vi "ComparaDataUART.vi"(8 "error in (no error)":errorcluster, 10 "StringIN":string, 11 "XuLyStringUART in":refnum<class "XuLyStringUART.lvclass">) -> (0 "error out":errorcluster, 3 "XuLyStringUART out":refnum<class "XuLyStringUART.lvclass">)   [LabVIEW 2017, in "LibraryGcode.lvlib" / "XuLyStringUART.lvclass"]
uses:
  XuLyStringUART.lvclass
  control/UartTypeDataGet.ctl
  controls/state_board_control.ctl
  XuLyStringUART.lvclass/XuLyStringUART.ctl
  control/UartStatusBusy.ctl
panel:
  out "outPOS":T1
  out "OUTCONFIG":T2
  out "Return State 2":T3=enum."Echo"
  in  "error IN":errorcluster
  out "error out 2":errorcluster
  in  "String IN":string
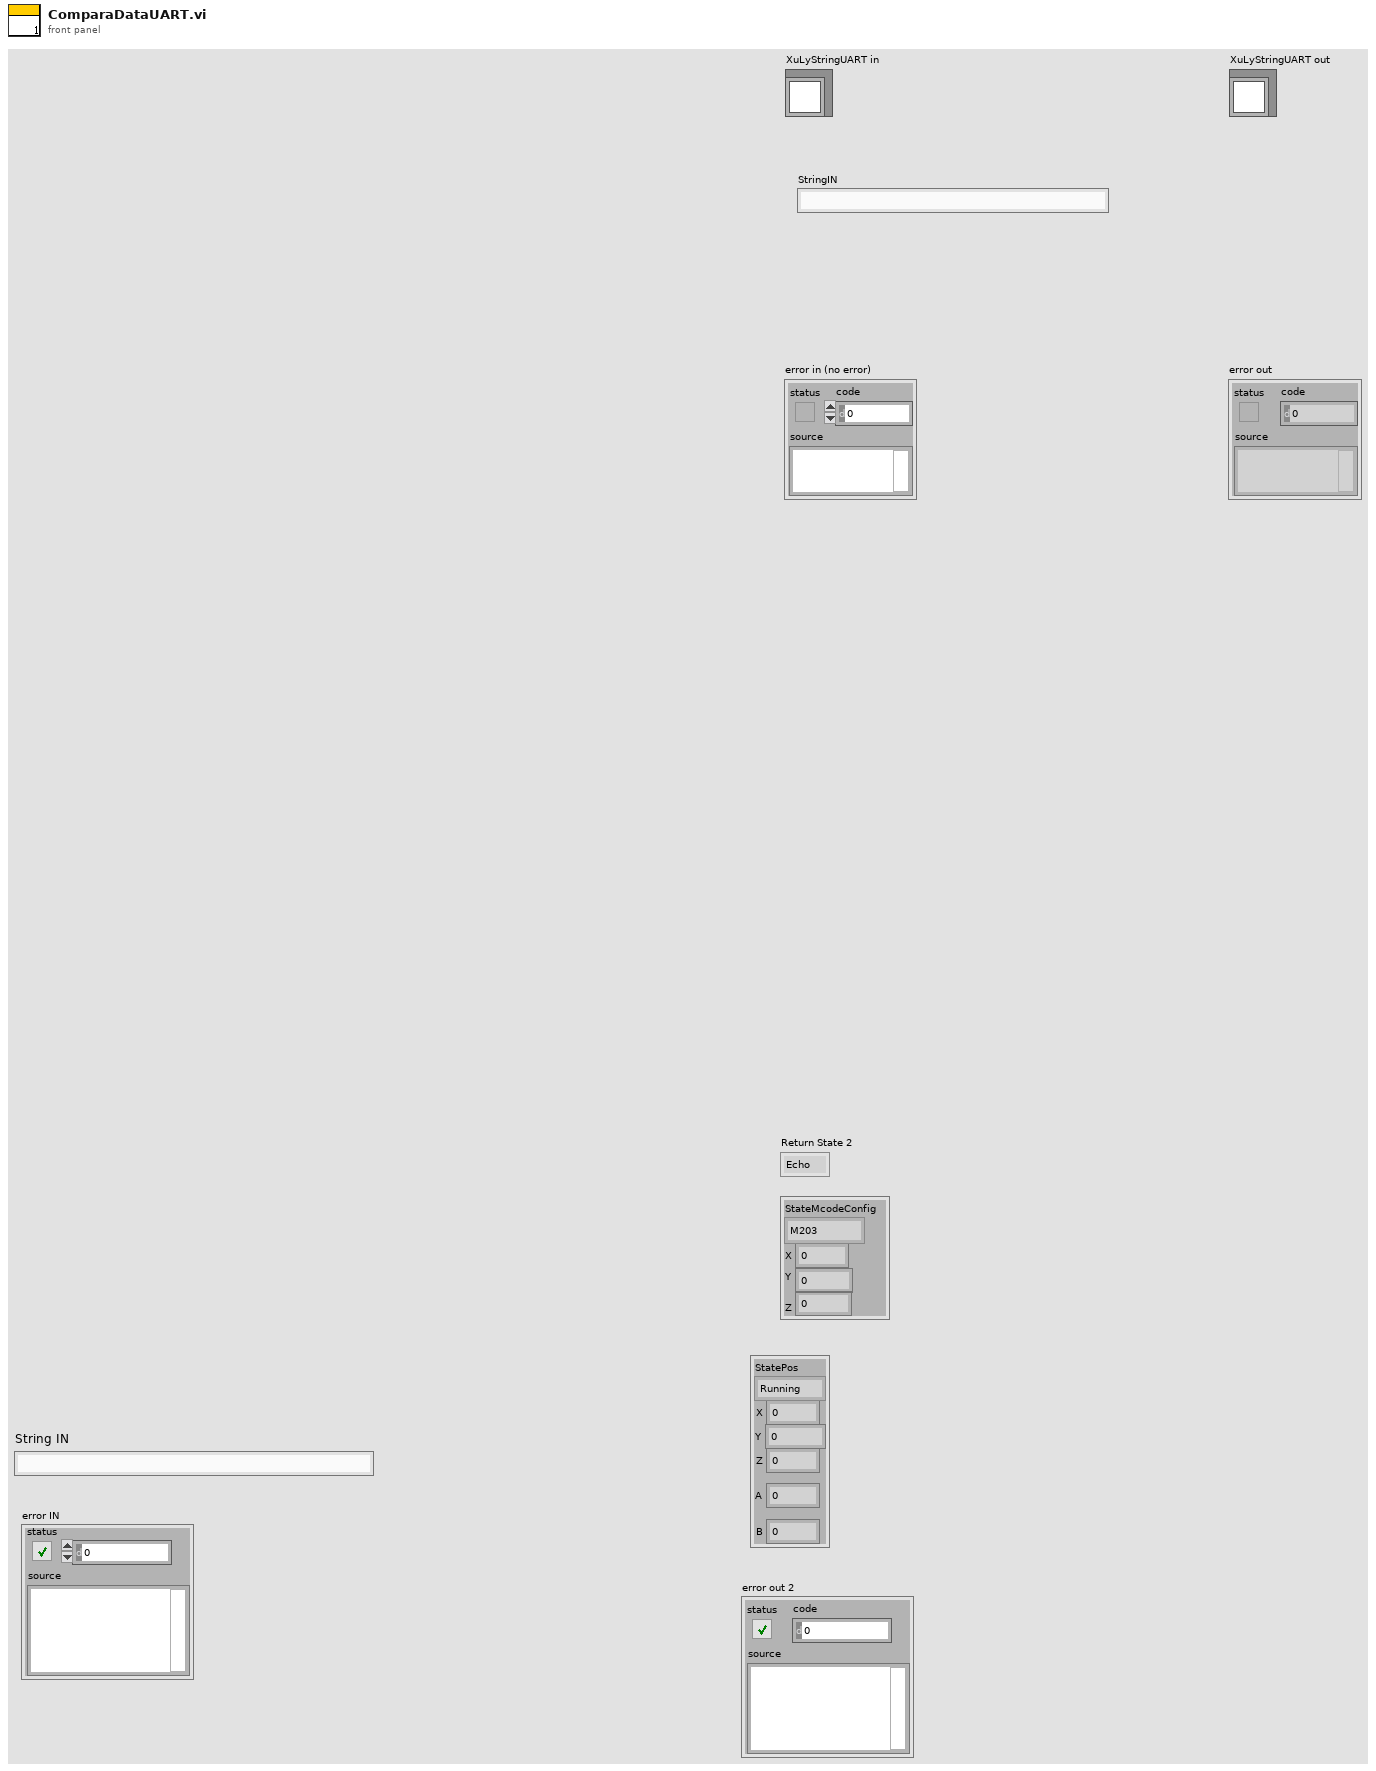
[diagram p1: front panel]
types:
  T1 = cluster{"StatePos":enum16{"Running", "Waiting", "Pos", "IDLE"}, "X":dbl, "Z":dbl, "Y":dbl, "A":dbl, "B":dbl}
  T2 = cluster{"StateMcodeConfig":enum16{"M203", "M201", "M92", "M3001", "M204"}, "X":dbl, "Y":dbl, "Z":dbl}
  T3 = typedef "UartTypeDataGet.ctl" = enum16{"Pos", "Config", "Echo", "OK", "Step", "Error"}
  T4 = typedef "UartStatusBusy.ctl" = enum16{"Running", "Waiting", "Pos", "IDLE"}
  T5 = typedef "state_board_control.ctl" = enum16{"Running", "Waiting", "Pos", "IDLE"}
  T6 = cluster{"StateMcodeConfig":enum16{"M203", "M201", "M92", "M3001", "M204"}, dbl, dbl, dbl}
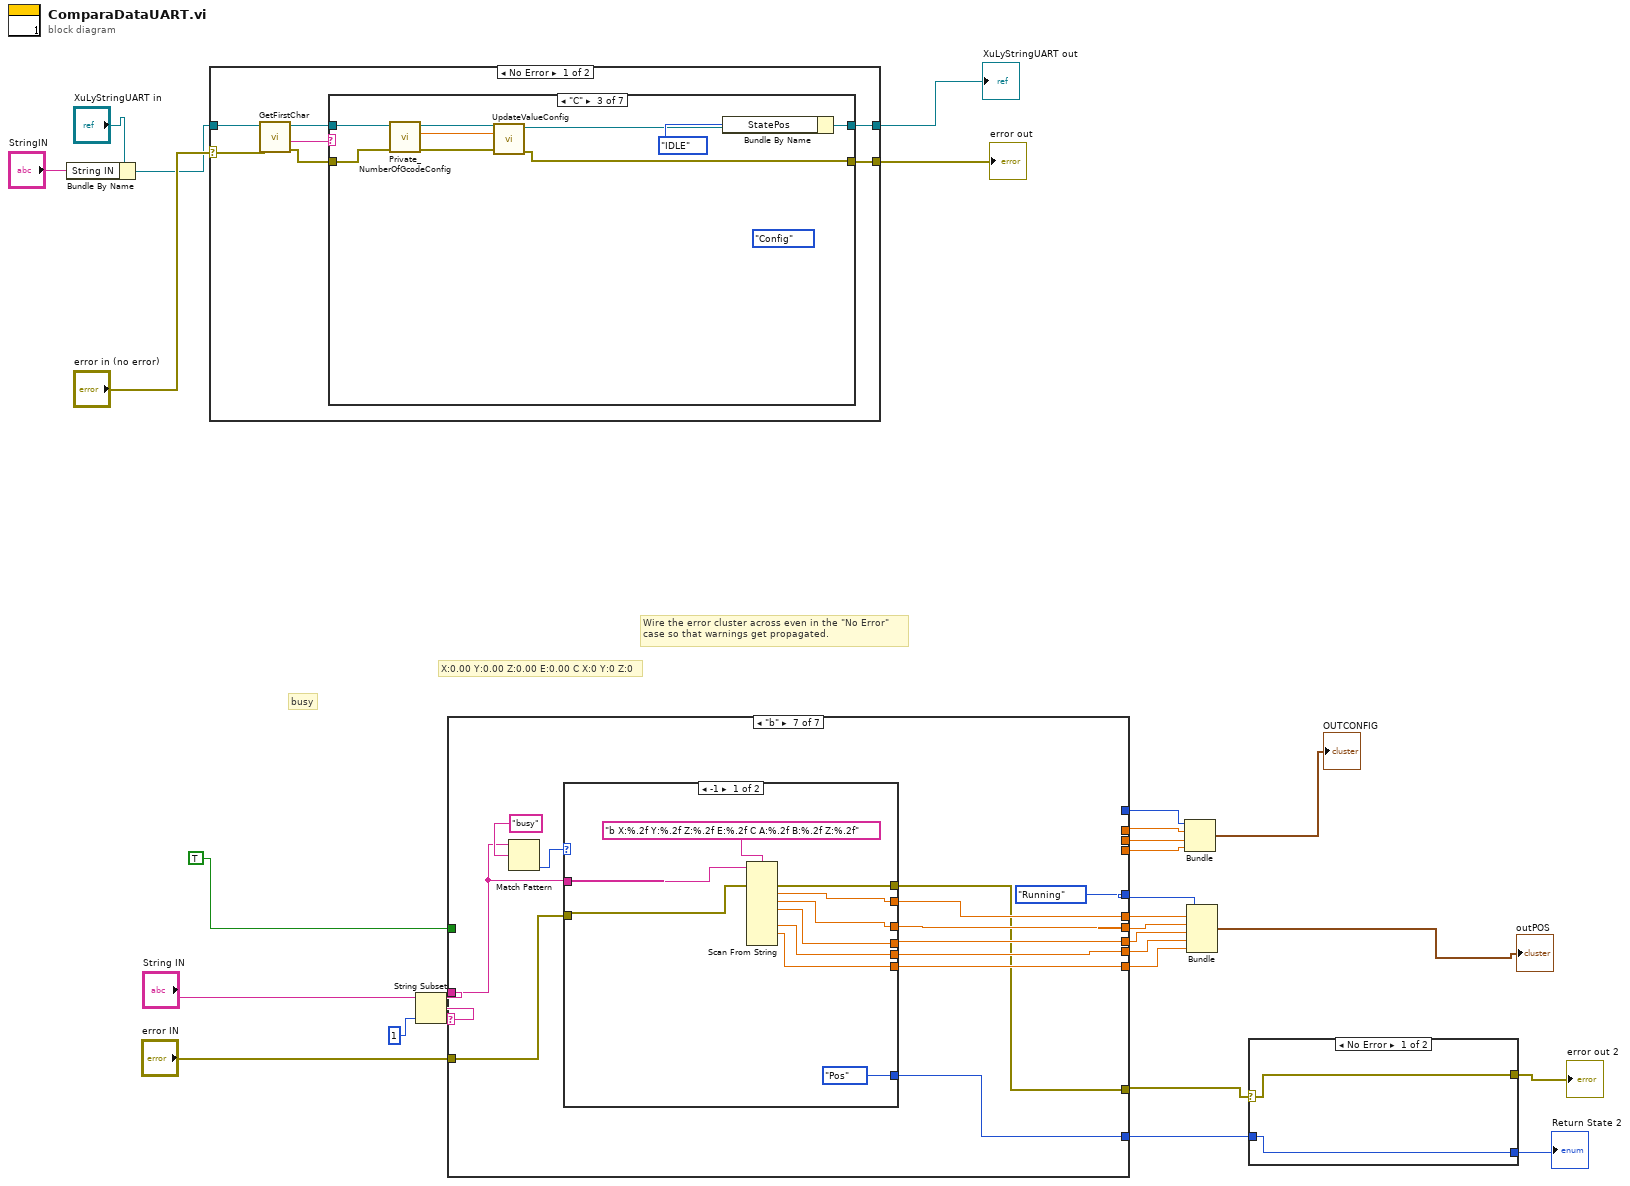
[diagram p0: block diagram]
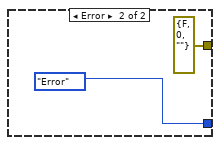
[diagram p2: hidden frame]
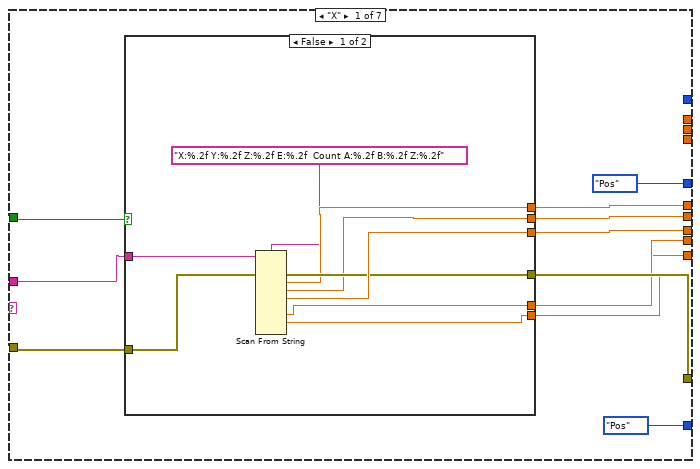
[diagram p3: hidden frame]
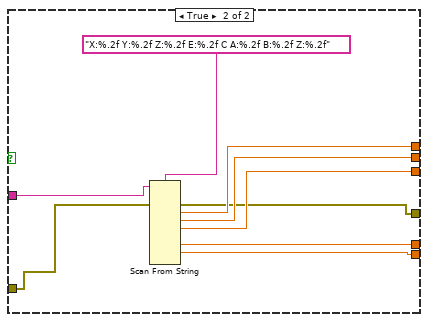
[diagram p4: hidden frame]
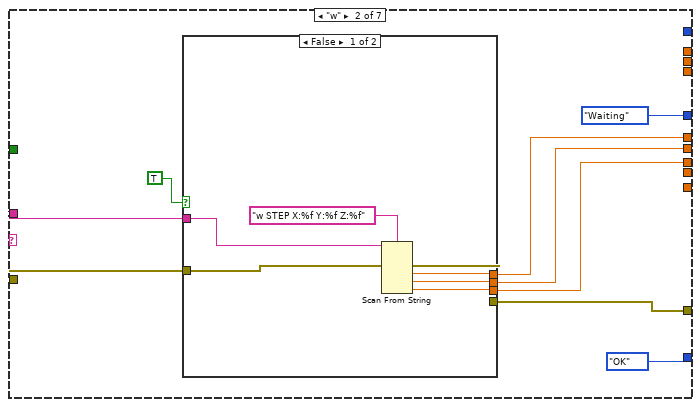
[diagram p5: hidden frame]
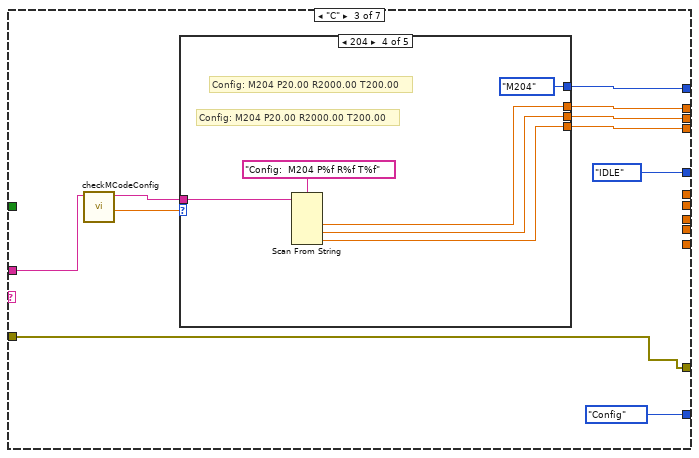
[diagram p7: hidden frame]
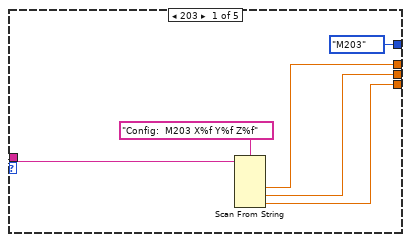
[diagram p8: hidden frame]
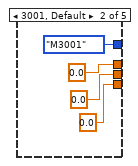
[diagram p9: hidden frame]
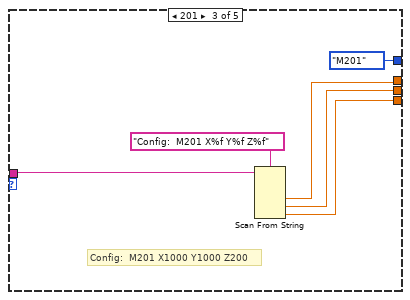
[diagram p10: hidden frame]
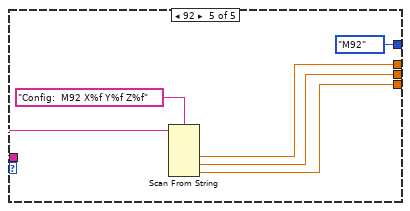
[diagram p11: hidden frame]
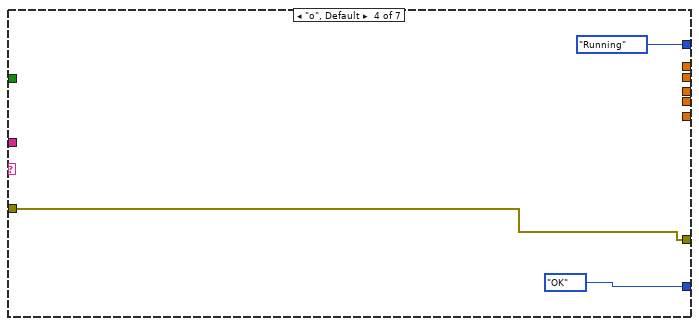
[diagram p12: hidden frame]
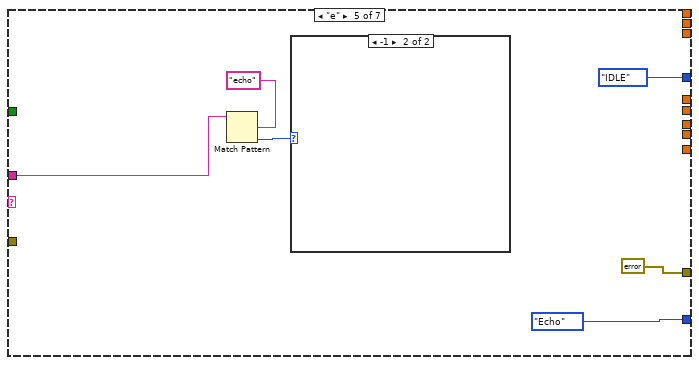
[diagram p13: hidden frame]
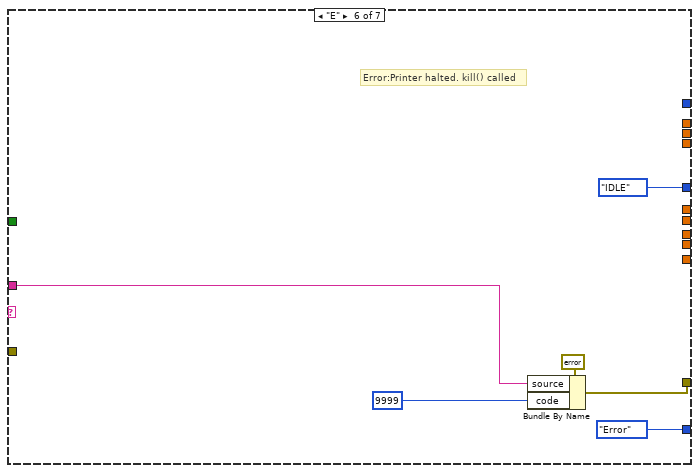
[diagram p15: hidden frame]
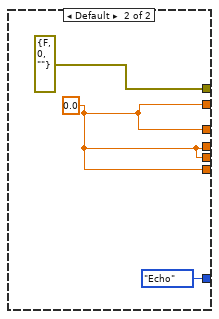
[diagram p16: hidden frame]
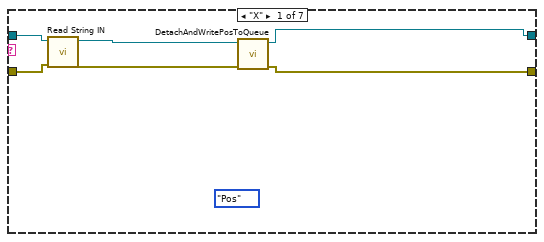
[diagram p17: hidden frame]
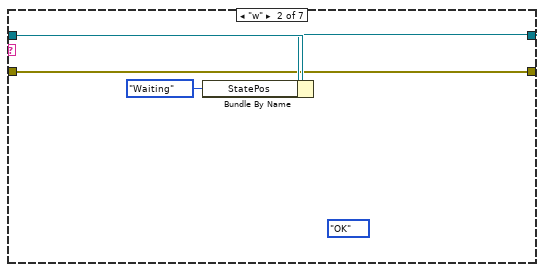
[diagram p18: hidden frame]
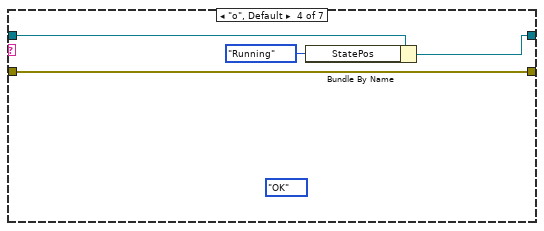
[diagram p19: hidden frame]
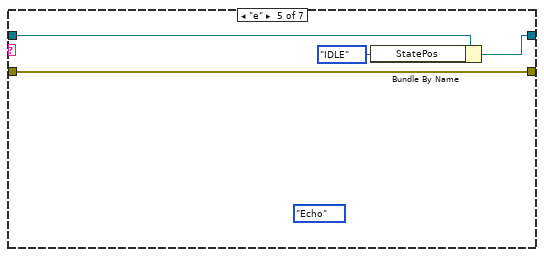
[diagram p20: hidden frame]
diagram:
  # "X:0.00 Y:0.00 Z:0.00 E:0.00 C X:0 Y:0 Z:0"
  # "busy"
  # "Wire the error cluster across even in the \"No Error\"\ncase so that warnings get propagated."
  n1 = Bundle By Name(cluster="XuLyStringUART in", "String IN"="StringIN") -> (w3:refnum<class "XuLyStringUART.lvclass">)
  n2 = case shown="No Error" "error in (no error)" {
    selector: "error in (no error)" -> [w30 w84]
    tunnel: [w28 w84] -> w26
    tunnel: [w34 w83] -> w25
    tunnel: w3 -> [w33 w83]
    frame No Error {
      n3 = call-dynamic "GetFirstChar.vi"("error in (no error)"=w30, "XuLyStringUART in"=w33) -> ("error out"=w29:errorcluster, "First Char"=w31:string, "XuLyStringUART out"=w32:refnum<class "XuLyStringUART.lvclass">)  [unwired: 7 in]
      n4 = case shown="\"C\"" w31 {
        tunnel: w29 -> [w39 w41 w52 w57 w59 _ w72]
        tunnel: [w38 w41 w48 w57 w59 w62 w74] -> w28
        tunnel: [w37 w43 w45 w54 w58 w64 w68] -> w34
        tunnel: w32 -> [w40 w44 w53 w56 w61 w66 w73]
        frame "X" {
          (unwired) UartTypeDataGet."Pos" ("Return State")
          n5 = call-dynamic "Read String IN.vi"("error in (no error)"=w39, "XuLyStringUART in"=w40) -> ("error out"=w35:errorcluster, "XuLyStringUART out"=w36:refnum<class "XuLyStringUART.lvclass">)  [unwired: 7 in, 1 out]
          n6 = call-dynamic "DetachAndWritePosToQueue.vi"("error in (no error)"=w35, "XuLyStringUART in"=w36) -> ("error out"=w38:errorcluster, "XuLyStringUART out"=w37:refnum<class "XuLyStringUART.lvclass">)  [unwired: 8 in]
        }
        frame "w" {
          (unwired) UartTypeDataGet."OK" ("Return State")
          n7 = Bundle By Name(cluster=w44, "StatePos"=UartStatusBusy."Waiting" ("outPOS.StatePos")) -> (w43:refnum<class "XuLyStringUART.lvclass">)
        }
        frame "C" {
          (unwired) UartTypeDataGet."Config" ("Return State")
          n8 = call-dynamic "Private_NumberOfGcodeConfig.vi"("error in (no error)"=w52, "XuLyStringUART in"=w53) -> ("error out"=w49:errorcluster, "McodeConfigNumber"=w50:dbl, "XuLyStringUART out"=w51:refnum<class "XuLyStringUART.lvclass">)  [unwired: 7 in]
          n9 = call-dynamic "UpdateValueConfig.vi"("error in (no error)"=w49, "McodeConfigNumber"=w50, "XuLyStringUART in"=w51) -> ("error out"=w48:errorcluster, "XuLyStringUART out"=w46:refnum<class "XuLyStringUART.lvclass">)  [unwired: 7 in]
          n10 = Bundle By Name(cluster=w46, "StatePos"=UartStatusBusy."IDLE" ("outPOS.StatePos")) -> (w45:refnum<class "XuLyStringUART.lvclass">)
        }
        frame "o", Default {
          (unwired) UartTypeDataGet."OK" ("Return State")
          n11 = Bundle By Name(cluster=w56, "StatePos"=UartStatusBusy."Running" ("outPOS.StatePos")) -> (w54:refnum<class "XuLyStringUART.lvclass">)
        }
        frame "e" {
          (unwired) UartTypeDataGet."Echo" ("Return State")
          n12 = Bundle By Name(cluster=w61, "StatePos"=UartStatusBusy."IDLE" ("outPOS.StatePos")) -> (w58:refnum<class "XuLyStringUART.lvclass">)
        }
        frame "E" {
          (unwired) UartTypeDataGet."Error" ("Return State")
          # "Error:Printer halted. kill() called"
          n13 = Bundle By Name(cluster=w66, "StatePos"=UartStatusBusy."IDLE" ("outPOS.StatePos")) -> (w64:refnum<class "XuLyStringUART.lvclass">)
          n14 = Bundle By Name(cluster=errorcluster {"status"=FALSE, "code"=0, "source"="REBOOT"} ("error IO"), "code"=9999) -> (w62:errorcluster)
        }
        frame "b" {
          n15 = call-dynamic "Read String IN.vi"("error in (no error)"=w72, "XuLyStringUART in"=w73) -> ("error out"=w70:errorcluster, "String IN"=w69:string, "XuLyStringUART out"=w71:refnum<class "XuLyStringUART.lvclass">)  [unwired: 7 in]
          n16 = Match Pattern(string=w69, regular expression="busy") -> (offset past match=w75:i32)  [unwired: 1 in, 3 out]
          n17 = case shown="-1" w75 {
            tunnel: w70 -> [w78 w81]
            tunnel: w71 -> [w80 w82]
            tunnel: [w79 w82] -> w68
            tunnel: [w77 w81] -> w74
            frame -1 {
              (unwired) UartTypeDataGet."Pos" ("Return State")
              n18 = call-dynamic "DetachAndWritePosToQueue.vi"("error in (no error)"=w78, "XuLyStringUART in"=w80) -> ("error out"=w77:errorcluster, "XuLyStringUART out"=w79:refnum<class "XuLyStringUART.lvclass">)  [unwired: 8 in]
            }
            frame Default {
              (unwired) UartTypeDataGet."Echo" ("Return State")
            }
          }
        }
      }
    }
    frame Error {
    }
  }
  "error out" <- w26
  "XuLyStringUART out" <- w25
  n19 = String Subset(string="String IN", length (rest)=1 ("length (rest)")) -> (substring=w10:string)  [unwired: 1 in]
  n20 = case shown="\"b\"" w10 {
    tunnel: [state_board_control."Pos" ("Enum") state_board_control."Waiting" ("Enum") state_board_control."IDLE" ("Enum") state_board_control."Running" ("Enum") enum16{"Running", "Waiting", "Pos", "IDLE"}."IDLE" ("Enum") state_board_control."IDLE" ("Enum") state_board_control."Running" ("Enum")] -> w23
    tunnel: [w91 w121 _ _ _ _ w191] -> w20
    tunnel: [w90 w120 _ _ _ _ w192] -> w19
    tunnel: [w95 w119 _ _ _ _ w193] -> w4
    tunnel: "error IN" -> [w94 w122 w131 w169 _ _ w190]
    tunnel: [w93 w118 w131 w169 errorcluster {"status"=FALSE, "code"=0, "source"=""} ("error IO") w181 w184] -> w14
    tunnel: [_ _ w139 _ _ _ _] -> w16
    tunnel: [_ _ w138 _ _ _ _] -> w17
    tunnel: [_ _ w137 _ _ _ _] -> w18
    tunnel: [_ _ w136 _ _ _ _] -> w15
    tunnel: [UartTypeDataGet."Pos" ("Return State") UartTypeDataGet."OK" ("Return State") UartTypeDataGet."Config" ("Return State") UartTypeDataGet."OK" ("Return State") UartTypeDataGet."Echo" ("Return State") UartTypeDataGet."Error" ("Return State") w189] -> w12
    tunnel: "String IN" -> [w85 w116 w133 _ w172 w178 w188]
    tunnel: TRUE -> [w88 _ _ _ _ _ _]
    tunnel: [w87 _ _ _ _ _ w186] -> w8
    tunnel: [w86 _ _ _ _ _ w185] -> w7
    frame "X" {
      n21 = case shown="False" w88 {
        tunnel: [w104 w109] -> w95
        tunnel: w94 -> [w103 w108]
        tunnel: [w102 w107] -> w93
        tunnel: [w101 w111] -> w91
        tunnel: [w100 w110] -> w90
        tunnel: w85 -> [w99 w112]
        tunnel: [w96 w106] -> w87
        tunnel: [w97 w105] -> w86
        frame False {
          n22 = Scan From String(format string="X:%.2f Y:%.2f Z:%.2f E:%.2f  Count A:%.2f B:%.2f Z:%.2f", input string=w99, error in=w103) -> (error out=w102:errorcluster, output 1=w101:dbl, output 2=w100:dbl, output 3=w104:dbl, output 5=w96:dbl, output 6=w97:dbl)  [unwired: 10 in, 2 out]
        }
        frame True {
          n23 = Scan From String(format string="X:%.2f Y:%.2f Z:%.2f E:%.2f C A:%.2f B:%.2f Z:%.2f", input string=w112, error in=w108) -> (error out=w107:errorcluster, output 1=w111:dbl, output 2=w110:dbl, output 3=w109:dbl, output 5=w106:dbl, output 6=w105:dbl)  [unwired: 10 in, 2 out]
        }
      }
    }
    frame "w" {
      n24 = case shown="False" TRUE {
        tunnel: w122 -> [w128 w130]
        tunnel: [w127 _] -> w121
        tunnel: [w126 _] -> w120
        tunnel: [w125 _] -> w119
        tunnel: [w124 w130] -> w118
        tunnel: w116 -> [w123 _]
        frame False {
          n25 = Scan From String(format string="w STEP X:%f Y:%f Z:%f", input string=w123, error in=w128) -> (error out=w124:errorcluster, output 1=w127:dbl, output 2=w126:dbl, output 3=w125:dbl)  [unwired: 4 in, 2 out]
        }
        frame True {
        }
      }
    }
    frame "C" {
      n26 = call "checkMCodeConfig.vi"("INPUT"=w133) -> ("MCODE"=w132:dbl, "OUTPUT"=w140:string)  [unwired: 9 in]
      n27 = case shown="204" w132 {
        tunnel: w140 -> [w145 _ w155 w161 w167]
        tunnel: [w144 0.0 w154 w159 w166] -> w139
        tunnel: [w143 0.0 w151 w158 w165] -> w138
        tunnel: [w142 0.0 w153 w157 w164] -> w137
        tunnel: [enum16{"M203", "M201", "M92", "M3001", "M204"}."M203" ("StateMcodeConfig") enum16{"M203", "M201", "M92", "M3001", "M204"}."M3001" ("StateMcodeConfig") enum16{"M203", "M201", "M92", "M3001", "M204"}."M201" ("StateMcodeConfig") enum16{"M203", "M201", "M92", "M3001", "M204"}."M204" ("StateMcodeConfig") enum16{"M203", "M201", "M92", "M3001", "M204"}."M92" ("StateMcodeConfig")] -> w136
        frame 203 {
          n28 = Scan From String(format string="Config:  M203 X%f Y%f Z%f", input string=w145) -> (output 1=w144:dbl, output 2=w143:dbl, output 3=w142:dbl)  [unwired: 5 in, 3 out]
        }
        frame 3001, Default {
        }
        frame 201 {
          # "Config:  M201 X1000 Y1000 Z200"
          n29 = Scan From String(format string="Config:  M201 X%f Y%f Z%f", input string=w155) -> (output 1=w154:dbl, output 2=w151:dbl, output 3=w153:dbl)  [unwired: 5 in, 3 out]
        }
        frame 204 {
          # "Config: M204 P20.00 R2000.00 T200.00"
          # "Config: M204 P20.00 R2000.00 T200.00"
          n30 = Scan From String(format string="Config:  M204 P%f R%f T%f", input string=w161) -> (output 1=w159:dbl, output 2=w158:dbl, output 3=w157:dbl)  [unwired: 5 in, 3 out]
        }
        frame 92 {
          n31 = Scan From String(format string="Config:  M92 X%f Y%f Z%f", input string=w167) -> (output 1=w166:dbl, output 2=w165:dbl, output 3=w164:dbl)  [unwired: 5 in, 3 out]
        }
      }
    }
    frame "o", Default {
    }
    frame "e" {
      n32 = Match Pattern(string=w172, regular expression="echo") -> (offset past match=w176:i32)  [unwired: 1 in, 3 out]
      n33 = case shown="-1" w176 {
        frame Default {
        }
        frame -1 {
        }
      }
    }
    frame "E" {
      # "Error:Printer halted. kill() called"
      n34 = Bundle By Name(cluster=errorcluster {"status"=FALSE, "code"=0, "source"="REBOOT"} ("error IO"), "source"=w178, "code"=9999) -> (w181:errorcluster)
    }
    frame "b" {
      n35 = Match Pattern(string=w188, regular expression="busy") -> (offset past match=w194:i32)  [unwired: 1 in, 3 out]
      n36 = case shown="-1" w194 {
        tunnel: w190 -> [w205 _]
        tunnel: [w204 errorcluster {"status"=FALSE, "code"=0, "source"=""} ("error IO")] -> w184
        tunnel: [w200 w206] -> w192
        tunnel: [w199 w206] -> w191
        tunnel: [w201 w206] -> w193
        tunnel: w188 -> [w203 _]
        tunnel: [UartTypeDataGet."Pos" ("Return State") UartTypeDataGet."Echo" ("Return State")] -> w189
        tunnel: [w196 w206] -> w186
        tunnel: [w197 w206] -> w185
        frame -1 {
          n37 = Scan From String(format string="b X:%.2f Y:%.2f Z:%.2f E:%.2f C A:%.2f B:%.2f Z:%.2f", input string=w203, error in=w205) -> (error out=w204:errorcluster, output 1=w199:dbl, output 2=w200:dbl, output 3=w201:dbl, output 5=w196:dbl, output 6=w197:dbl)  [unwired: 10 in, 2 out]
        }
        frame Default {
          w206 = 0.0
        }
      }
    }
  }
  n38 = Bundle("StateMcodeConfig"=w15, w16, w17, w18) -> (→"OUTCONFIG":T6)  [unwired: 1 in]
  n39 = Bundle("Enum"=w23, w20, w19, w4, w8, w7) -> (→"outPOS":cluster{"Enum":T5, dbl, dbl, dbl, dbl, dbl})  [unwired: 1 in]
  n40 = case shown="No Error" w14 {
    selector: w14 -> [w210 _]
    tunnel: [w210 errorcluster {"status"=FALSE, "code"=0, "source"=""} ("error IO")] -> w22
    tunnel: w12 -> [w209 _]
    tunnel: [w209 UartTypeDataGet."Error" ("Return State")] -> w13
    frame No Error {
    }
    frame Error {
    }
  }
  "error out 2" <- w22
  "Return State 2" <- w13
